vi "Bad Idea Globals.vi"() -> ()   [LabVIEW 2023]
panel:
  out "Is Running?":bool
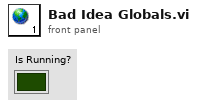
[diagram p1: front panel]
diagram:
